vi "Wrapper.vi"(8 "error in (no error)":errorcluster, 10 "setpoint":dbl, 11 "loop period update":refnum<notifier>) -> (0 "error out":errorcluster, 3 "output":dbl)   [LabVIEW 2024, in "PID Controller.lvlib" / "PID Controller.lvclass"]
uses:
  PID Controller.lvclass
  <vilib>/addons/control/pid/pid.llb/PID (DBL).vi
  PID Controller.lvclass/PID Controller.ctl
  <vilib>/addons/control/pid/NI_PID_pid.lvlib
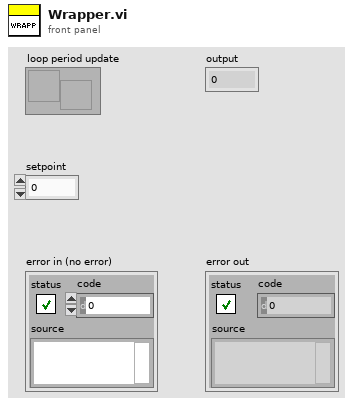
[diagram p1: front panel]
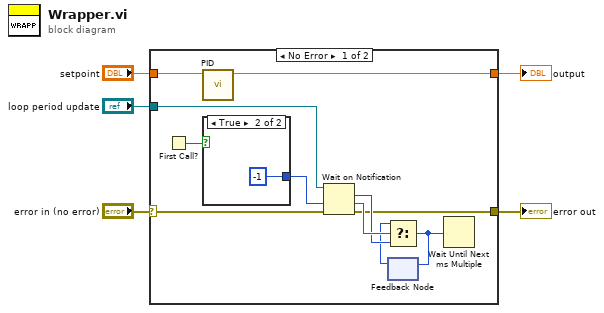
[diagram p0: block diagram]
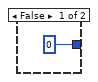
[diagram p2: hidden frame]
diagram:
  n1 = case shown="No Error" "error in (no error)" {
    selector: "error in (no error)" -> [w7 w19]
    tunnel: [w6 w19] -> w4
    tunnel: "loop period update" -> [w12 _]
    tunnel: [w9 _] -> w2
    tunnel: "setpoint" -> [w8 _]
    frame No Error {
      n2 = First Call?() -> (First Call?: T/F=w16:bool)
      n3 = call-poly <vilib>:"PID.vi"("setpoint"=w8) -> ("output"=w9:dbl)  [unwired: 9 in, 1 out]
      n4 = case shown="True" w16 {
        tunnel: [0 ("timeout in ms (-1)") -1 ("timeout in ms (-1)")] -> w15
        frame False {
        }
        frame True {
        }
      }
      n5 = Wait on Notification(notifier=w12, timeout in ms (-1)=w15, error in (no error)=w7) -> (notification=w13:u32, timed out?=w14:bool, error out=w6:errorcluster)  [unwired: 1 in, 1 out]
      n6 = feedback #1() -> (w10:u32)  [unwired: 1 in]
      n7 = Select(t=w10, s=w14, f=w13) -> (s? t:f=w11:u32)
      n8 = feedback-in #1(w11) -> ()
      n9 = Wait Until Next ms Multiple(millisecond multiple=w11) -> ()  [unwired: 1 out]
    }
    frame Error {
    }
  }
  "error out" <- w4
  "output" <- w2
